vi "read N samples N channels.vi"(8 "error in (no error)":errorcluster, 11 "CompactDAQ in":refnum<class "CompactDAQ.lvclass">) -> (0 "error out":errorcluster, 2 "data":dbl[][](array[numeric]) format="%0.2f", 3 "CompactDAQ out":refnum<class "CompactDAQ.lvclass">)   [LabVIEW 2017, in "CompactDAQ.lvclass"]
uses:
  CompactDAQ.lvclass
  \\Mac\Home/Documents/MAL-Framework/user.lib/Common Components/Hardware/Hardware.lvclass
  <userlib>/Common Components/Hardware/Hardware.lvclass/Hardware.ctl
  CompactDAQ.lvclass/CompactDAQ.ctl
  <vilib>/DAQmx/read.llb/DAQmx Read (Analog 2D DBL NChan NSamp).vi
  <vilib>/DAQmx/miscellaneous.llb/DAQmx Fill In Error Info.vi
  <userlib>/Common Components/Hardware/Hardware.lvclass
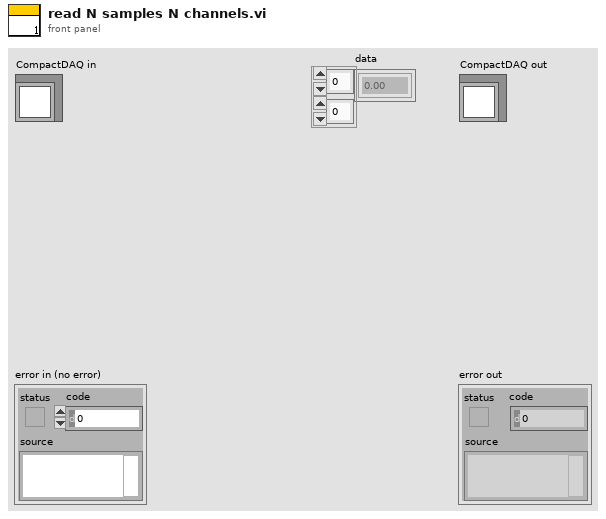
[diagram p1: front panel]
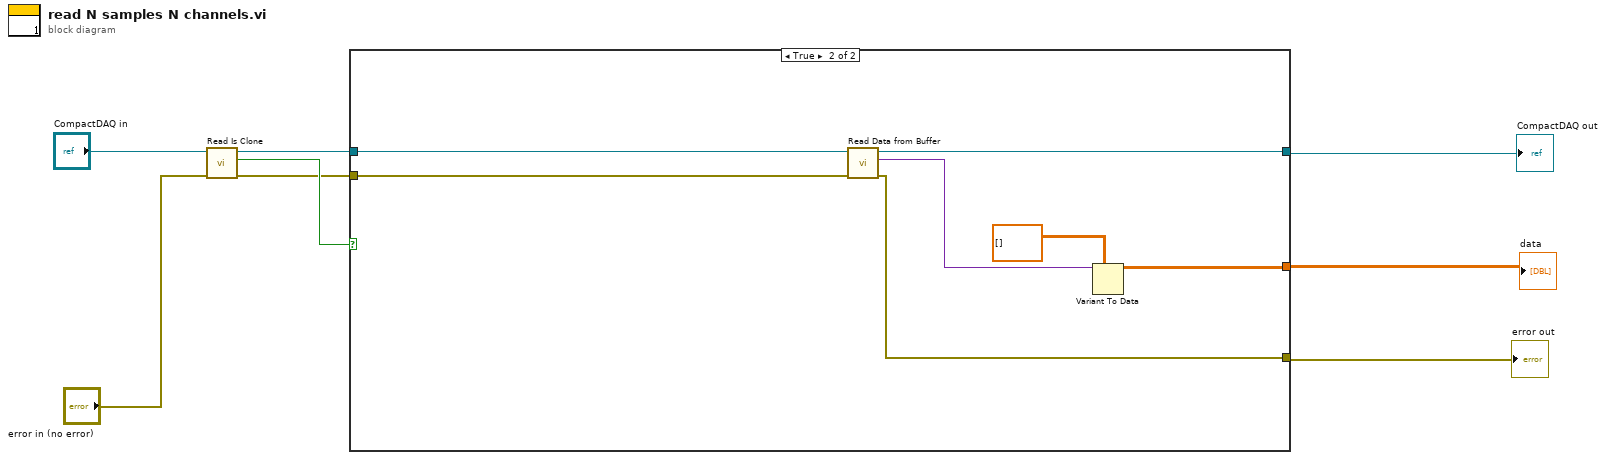
[diagram p0: block diagram]
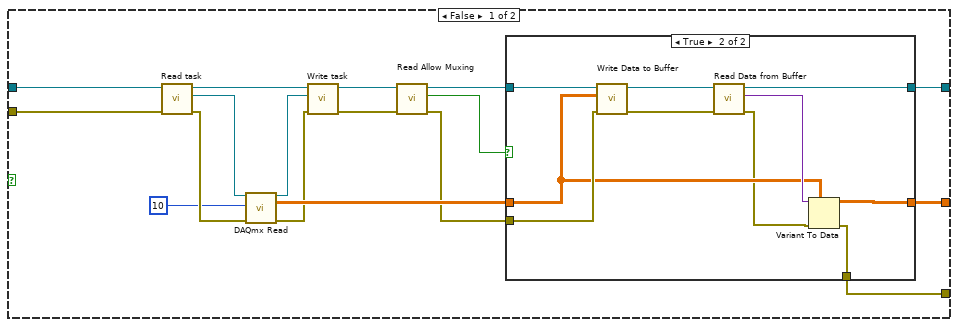
[diagram p2: hidden frame]
diagram:
  n1 = call <userlib>:"Read Is Clone.vi"("error in (no error)"="error in (no error)", "Hardware in"="CompactDAQ in") -> ("error out"=w2:errorcluster, "Is Clone?"=w4:bool, "Hardware out"=w5:refnum<class "CompactDAQ.lvclass">)  [unwired: 7 in]
  n2 = case shown="True" w4 {
    tunnel: w5 -> [w24 w45]
    tunnel: [w21 w44] -> w8
    tunnel: [w19 w40] -> w1
    tunnel: [w18 w42] -> w7
    tunnel: w2 -> [w14 w43]
    frame False {
      n3 = call "Read task.vi"("error in (no error)"=w14, "CompactDAQ in"=w24) -> ("error out"=w13:errorcluster, "task"=w25:refnum<k21>, "CompactDAQ out"=w22:refnum<class "CompactDAQ.lvclass">)  [unwired: 7 in]
      n4 = call-poly <vilib>:"DAQmx Read.vi"("task/channels in"=w25, "number of samples per channel"=10, "error in"=w13) -> ("task out"=w23:refnum<k21>, "data"=w20:dbl[][], "error out"=w11:errorcluster)  [unwired: 10 in]
      n5 = call "Write task.vi"("error in (no error)"=w11, "task"=w23, "CompactDAQ in"=w22) -> ("error out"=w12:errorcluster, "CompactDAQ out"=w17:refnum<class "CompactDAQ.lvclass">)  [unwired: 7 in]
      n6 = call <userlib>:"Read Allow Muxing.vi"("error in (no error)"=w12, "Hardware in"=w17) -> ("error out"=w10:errorcluster, "Allow Muxing"=w15:bool, "Hardware out"=w16:refnum<class "CompactDAQ.lvclass">)  [unwired: 7 in]
      n7 = case shown="True" w15 {
        tunnel: [w27 w37] -> w21
        tunnel: w10 -> [w26 w35]
        tunnel: w20 -> [w28 w33]
        tunnel: [w28 w32] -> w19
        tunnel: [w26 w30] -> w18
        tunnel: w16 -> [w27 w29]
        frame False {
        }
        frame True {
          n8 = call <userlib>:"Write Data to Buffer.vi"("error in (no error)"=w35, "Data"=w33, "Hardware in"=w29) -> ("error out"=w36:errorcluster, "Hardware out"=w38:refnum<class "CompactDAQ.lvclass">)  [unwired: 7 in]
          n9 = call <userlib>:"Read Data from Buffer.vi"("error in (no error)"=w36, "Hardware in"=w38) -> ("error out"=w31:errorcluster, "Variant"=w34:variant, "Hardware out"=w37:refnum<class "CompactDAQ.lvclass">)  [unwired: 7 in]
          n10 = Variant To Data(error in=w31, type=w33, Variant=w34) -> (data=w32:dbl[][], error out=w30:errorcluster)
        }
      }
    }
    frame True {
      n11 = call <userlib>:"Read Data from Buffer.vi"("error in (no error)"=w43, "Hardware in"=w45) -> ("error out"=w42:errorcluster, "Variant"=w41:variant, "Hardware out"=w44:refnum<class "CompactDAQ.lvclass">)  [unwired: 7 in]
      n12 = Variant To Data(type=dbl[][] [] ("data"), Variant=w41) -> (data=w40:dbl[][])  [unwired: 1 in, 1 out]
    }
  }
  "error out" <- w7
  "CompactDAQ out" <- w8
  "data" <- w1
